vi "Control Arm wrist with PID 2.vi"(10 "stop":bool) -> (2 "motorStop":bool, 3 "busy":bool)   [LabVIEW 2015]
uses:
  <vilib>/myRIO/Common/Instrument Driver Framework/myRIO v1.0/Encoder/typedefs/Encoder Signal Mode.ctl
  <vilib>/myRIO/Instrument Drivers/Onboard IO/Encoder/typedefs/Encoder Reference.ctl
  <vilib>/myRIO/Common/Instrument Driver Framework/Utilities/typedefs/myRIO Generic Hardware Reference.ctl
  <vilib>/myRIO/Common/Instrument Driver Framework/Utilities/typedefs/Hardware Version Enum.ctl
  <vilib>/myRIO/Common/Instrument Driver Framework/Utilities/typedefs/myRIO v1.0 Reference.ctl
  <vilib>/myRIO/Common/Instrument Driver Framework/Utilities/typedefs/Generic FPGA Reference.ctl
  <vilib>/myRIO/Common/Instrument Driver Framework/myRIO v1.0/Encoder/typedefs/Encoder Channels Enum.ctl
  <vilib>/myRIO/Common/Instrument Driver Framework/myRIO v1.0/Encoder/typedefs/Encoder Configuration v1.0.ctl
  <vilib>/userdefined/High Color/nirio_resource_hc.ctl
  <vilib>/myRIO/Common/Instrument Driver Framework/Utilities/vis/Is FPGA Ref Available.vi
  <vilib>/myRIO/Common/Instrument Driver Framework/myRIO v1.0/Encoder/vis/myRIO v1.1 Open Encoder.vi
  <vilib>/myRIO/Instrument Drivers/Onboard IO/Encoder/vis/Read.vi
  <vilib>/myRIO/Common/Instrument Driver Framework/Utilities/vis/Validate Channels.vi
  <vilib>/myRIO/Common/Instrument Driver Framework/myRIO v1.0/Encoder/vis/myRIO v1.0 Reserve Encoder.vi
  <vilib>/myRIO/Common/Instrument Driver Framework/myRIO v1.0/Encoder/vis/myRIO v1.0 Build MUX Configuration Encoder.vi
  <vilib>/myRIO/Common/Instrument Driver Framework/myRIO v1.0/Resource Manager/vis/myRIO v1.0 Reserve Channel List.vi
  <vilib>/myRIO/Common/Instrument Driver Framework/myRIO v1.0/Resource Manager/vis/myRIO v1.0 Create Configuration List.vi
  <vilib>/myRIO/Common/Instrument Driver Framework/myRIO v1.0/Resource Manager/vis/myRIO v1.0 Reserve Channel.vi
  <vilib>/myRIO/Common/Instrument Driver Framework/myRIO v1.0/Resource Manager/vis/myRIO v1.0 Unreserve Channel.vi
  <vilib>/myRIO/Common/Instrument Driver Framework/myRIO v1.0/Resource Manager/vis/myRIO v1.0 Build Mutex Name.vi
  Global Angle.vi
  <vilib>/Utility/VariantDataType/GetNumericInfo.vi
  <vilib>/Utility/error.llb/Error Cluster From Error Code.vi
  <vilib>/myRIO/Common/Instrument Driver Framework/myRIO v1.0/myRIO v1.1 Open.vi
  <vilib>/myRIO/Common/Instrument Driver Framework/Utilities/vis/IO Manager.vi
  <vilib>/myRIO/Common/Instrument Driver Framework/Utilities/vis/Configuration Manager.vi
  <vilib>/myRIO/Common/Instrument Driver Framework/myRIO v1.0/Resource Manager/vis/myRIO v1.0 Configure IO.vi
  <vilib>/myRIO/Common/Instrument Driver Framework/myRIO v1.0/myRIO v1.0 Close.vi
  <vilib>/myRIO/Common/Instrument Driver Framework/myRIO v1.0/Encoder/vis/myRIO v1.0 Configure Encoder.vi
  <vilib>/myRIO/Common/Instrument Driver Framework/myRIO v1.0/Encoder/vis/myRIO v1.0 Read Encoder.vi
  <vilib>/myRIO/Express VI/Onboard IO/Encoder/Encoder Express VI.xnode
  <vilib>/myRIO/Instrument Drivers/Onboard IO/Encoder/vis/myRIO Encoder Open.xnode
  <vilib>/myRIO/Common/Instrument Driver Framework/myRIO v1.0/Encoder/typedefs/Encoder Count Direction Enum.ctl
  <vilib>/myRIO/Instrument Drivers/Onboard IO/Encoder/Encoder.lvlib
panel:
  out "NaNBit":bool
  in  "Pd":dbl
  in  "Pi":dbl
  in  "Pp":dbl
  out "Wrist Angle":dbl(slide) scale=-300.0..500.0
  out "input Angles":dbl
  out "output":i32
  out "differential":i32
  out "error":i32
  out "input Rotations":dbl
  out "lastError":dbl
  out "Counter Value":i32
  # "Arm Wrist  Control"
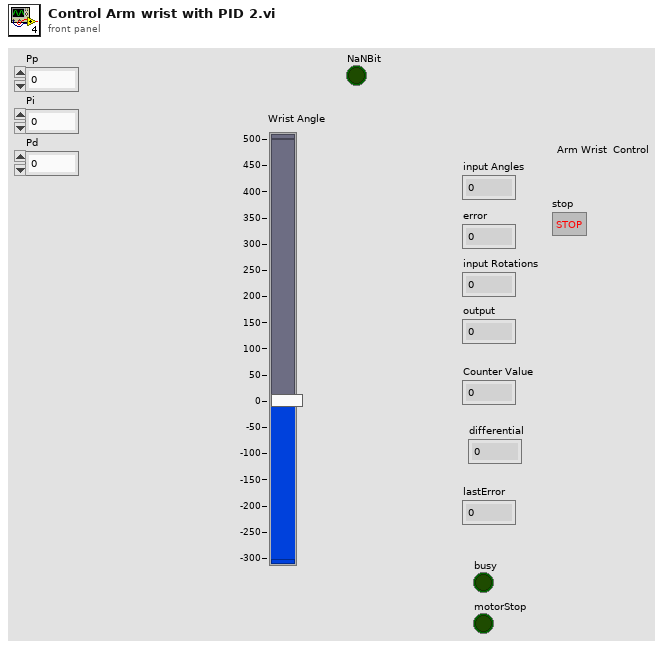
[diagram p1: front panel]
types:
  T1 = typedef "Encoder.lvlib/Encoder Reference.ctl" = cluster{"myRIO Reference":T2, "Encoder Channels Enum":T6}
  T2 = typedef "myRIO Generic Hardware Reference.ctl" = cluster{"myRIO Model":T3, "myRIO Hardware Reference":T4}
  T3 = typedef "Hardware Version Enum.ctl" = enum16{"Unknown", "myRIO-1900", "myRIO-1950", "roboRIO"}
  T4 = typedef "myRIO v1.0 Reference.ctl" = cluster{"Generic FPGA Reference":T5, "Allow multiple opens":bool}
  T5 = typedef "Generic FPGA Reference.ctl" = refnum<k20>
  T6 = typedef "Encoder Channels Enum.ctl" = enum16{"Not Connected", "C/ENC0", "C/ENC1", "A/ENC", "B/ENC", "DIO/ENC0", "DIO/ENC1", "DIO/ENC2", "DIO/ENC3", "DIO/ENC4"}
  T7 = typedef "Encoder Signal Mode.ctl" = enum16{"Quadrature phase signal", "Step and direction signal"}
  T8 = typedef "nirio_resource_hc.ctl" = tag
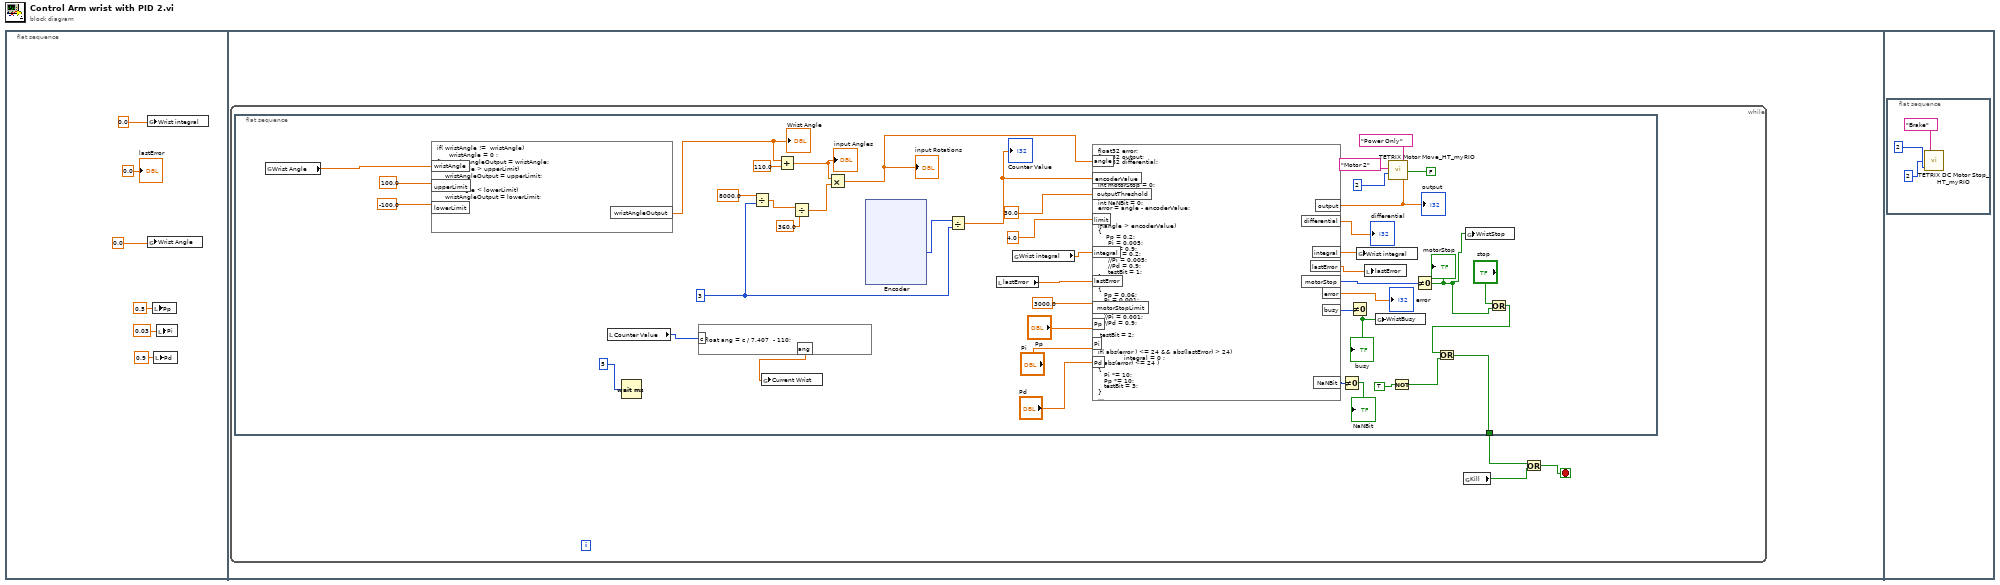
[diagram p0: block diagram]
diagram:
  n1 = flat-sequence {
    frame #0 {
      n2 = global write "Global Angle.vi" "Wrist integral"(0.0 ("integral")) -> ()
      n3 = global write "Global Angle.vi" "Wrist Angle"(0.0 ("angle")) -> ()
      n4 = local write "Pp"(0.5 ("Pp")) -> ()
      n5 = local write "Pd"(0.9 ("Pd")) -> ()
      n6 = local write "Pi"(0.03 ("Pi")) -> ()
      "lastError" <- 0.0 ("lastError")
    }
    frame #1 {
      n7 = while {
        stop <- w7 stop-if-true
        n8 = flat-sequence {
          tunnel: [w36] -> w9
          frame #0 {
            w20 = 3 ("y")
            n9 = global read "Global Angle.vi" "Wrist Angle"() -> (w17:dbl)
            n10 = formula code="if( wristAngle !=  wristAngle)\n      wristAngle = 0 ;\nfloat wristAngleOutput = wristAngle;\nif(wristAngle > upperLimit)\n    wristAngleOutput = upperLimit;\n\nif(wristAngle < lowerLimit)\n    wristAngleOutput = lowerLimit;"("wristAngle"=w17, "upperLimit"=100.0 ("input variable"), "lowerLimit"=-100.0 ("input variable")) -> ("wristAngleOutput"=w23:dbl)
            "Wrist Angle" <- w23
            n11 = local read "Counter Value"() -> (w11:i32)
            n12 = Wait (ms)(milliseconds to wait=u32 5) -> ()  [unwired: 1 out]
            n13 = formula code="float ang = c / 7.407  - 110;"("c"=w11) -> ("ang"=w10:dbl)
            n14 = Divide(x=8000.0, y=w20) -> (x/y=w21:dbl)
            n15 = global write "Global Angle.vi" "Current Wrist"(w10) -> ()
            n16 = Add(x=w23, y=110.0) -> (x+y=w31:dbl)
            "input Angles" <- w31
            n17 = Divide(x=w21, y=360.0) -> (x/y=w34:dbl)
            n18 = Multiply(x=w31, y=w34) -> (x*y=w32:dbl)
            "input Rotations" <- w32
            n19 = xnode "Encoder"() -> ("Counter Value"=w47:i32)  [unwired: 2 in, 3 out]
            n20 = Divide(x=w47, y=w20) -> (x/y=w46:dbl)
            "Counter Value" <- w46
            n21 = local read "lastError"() -> (w50:dbl)
            n22 = global read "Global Angle.vi" "Wrist integral"() -> (w28:dbl)
            n23 = formula code="float32 error;\nfloat32 output;\nfloat32 differential;\n\n\n\nint motorStop = 0;\nint busy = 1;\nint testBit = 0;\nint NaNBit = 0;\nerror = angle - encoderValue;\n\n\nif(angle > encoderValue)\n{\n    Pp = 0.2;\n     Pi = 0.005;\n     Pd = 0.9;\n     //Pp = 0.2;\n     //Pi = 0.005;\n     //Pd = 0.9;\n     testBit = 1;\n}\nelse\n{\n   Pp = 0.06;\n   Pi = 0.001;\n   Pd = 0.9;\n   //Pp = 0.06;\n   //Pi = 0.001;\n   //Pd = 0.9;\n    \n testBit = 2;\n}\n\nif( abs(error ) <= 24 && abs(lastError) > 24) \n             integral = 0 ;\nif(abs(error) <= 24 )\n{\n   Pi *= 10;\n   Pp *= 10;\n   testBit = 3;\n}\n        \nintegral +=Pi*error;\ndifferential = Pd*(error - lastError);\n\n// P parameter:\noutput = error *Pp;\n// I parameter:\noutput += integral;\n// D parameter:\noutput += differential;\n\nlastError = error;\n\nif( abs(error) <= limit)\n{\n     output = 0;\n      integral = 0;\n      busy = 0;\n}\n \n\nif( abs(output) >= outputThreshold)\n {\n      if(output > 0)\n                   output = outputThreshold;\n      else \n                  output = -1*outputThreshold;\n}\n\nif(abs(integral) >= motorStopLimit &&  abs(error) <= 24)\n      motorStop = 1;"("angle"=w32, "encoderValue"=w46, "outputThreshold"=30.0 ("input variable"), "limit"=4.0 ("input variable"), "integral"=w28, "lastError"=w50, "motorStopLimit"=3000.0 ("input variable"), "Pp"="Pp", "Pi"="Pi", "Pd"="Pd") -> ("output"=w40:sgl, "integral"=w29:dbl, "lastError"=w49:dbl, "error"=→"error":sgl, "motorStop"=w44:i32, "differential"=→"differential":sgl, "busy"=w35:i32, "NaNBit"=w13:i32)
            "output" <- w40
            n24 = Not Equal To 0?(x=w13) -> (x != 0?=→"NaNBit":bool)
            n25 = Not Equal To 0?(x=w35) -> (x != 0?=w18:bool)
            "busy" <- w18
            n26 = global write "Global Angle.vi" "Wrist integral"(w29) -> ()
            n27 = local write "lastError"(w49) -> ()
            n28 = global write "Global Angle.vi" "WristBusy"(w18) -> ()
            n29 = call <vilib>:"TETRIX Motor Move_HT_myRIO.vi"("Power (-100 to 100)\n0 = Stop/Brake\n-128 = Stop/Coast"=w40, "Reverse? : T or F"=FALSE, "Control Mode"="Power Only", "Controller Daisy Chain Position: 1 - 4"=u8 2, "Select Channel"="Motor 2") -> ()  [unwired: 2 in, 1 out]
            n30 = Not(x=TRUE) -> (.not. x?=w37:bool)
            n31 = Not Equal To 0?(x=w44) -> (x != 0?=w19:bool)
            "motorStop" <- w19
            n32 = global write "Global Angle.vi" "WristStop"(w19) -> ()
            n33 = Or(x="stop", y=w19) -> (x .or. y?=w38:bool)
            n34 = Or(x=w38, y=w37) -> (x .or. y?=w36:bool)
          }
        }
        n35 = global read "Global Angle.vi" "Kill"() -> (w8:bool)
        n36 = Or(x=w9, y=w8) -> (x .or. y?=w7:bool)
      }
    }
    frame #2 {
      n37 = flat-sequence {
        frame #0 {
          n38 = call <vilib>:"TETRIX DC Motor Stop_HT_myRIO.vi"("Stop (Brake or Coast)"="Brake", "Motor Channel: (1 or 2)"=u8 2, "Controller Daisy Chain Position: 1 - 4"=u8 2) -> ()  [unwired: 1 in, 1 out]
        }
      }
    }
  }
